vi "sysexec.vi"   [LabVIEW 2014]
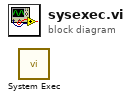
[diagram p0: block diagram]
diagram:
  n1 = call <vilib>:"System Exec.vi"() -> ()  [unwired: 8 in, 4 out]
